vi "piezoDoubleSync.vi"() -> ()   [LabVIEW 2017]
panel:
  in  "stop":bool
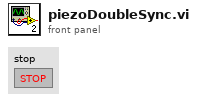
[diagram p1: front panel]
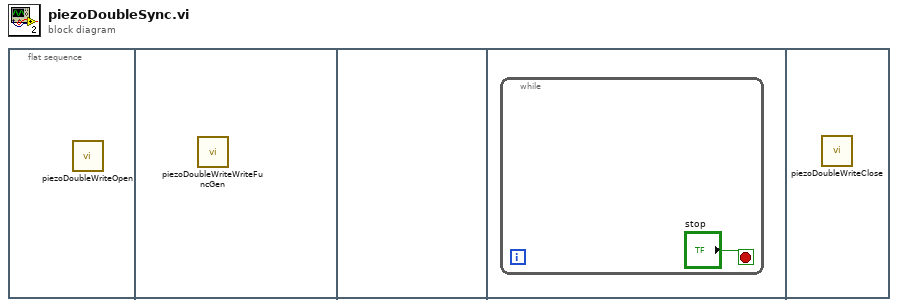
[diagram p0: block diagram]
diagram:
  n1 = flat-sequence {
    frame #0 {
      n2 = call "piezoDoubleWriteOpen.vi"() -> ()  [unwired: 2 in]
    }
    frame #1 {
      n3 = call "piezoDoubleWriteWriteFuncGen.vi"() -> ()  [unwired: 1 in, 1 out]
    }
    frame #2 {
    }
    frame #3 {
      n4 = while {
        stop <- "stop" stop-if-true
      }
    }
    frame #4 {
      n5 = call "piezoDoubleWriteClose.vi"() -> ()  [unwired: 1 in]
    }
  }
